vi "旧-试验模式表.vi"() -> ()   [LabVIEW 2013]
panel:
  in  "旧-试验模式表":string[](array[string])
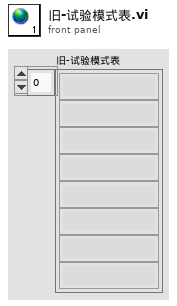
[diagram p1: front panel]
diagram:
